vi "CRYAPI Spliter Ref.vi"(0 "VI Refnum":refnum<vi>) -> (1 "Left/Upper":refnum<vi>, 2 "Right/Lower":refnum<vi>)   [LabVIEW 2013]
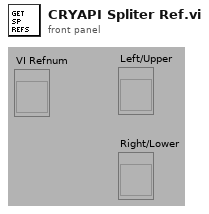
[diagram p1: front panel]
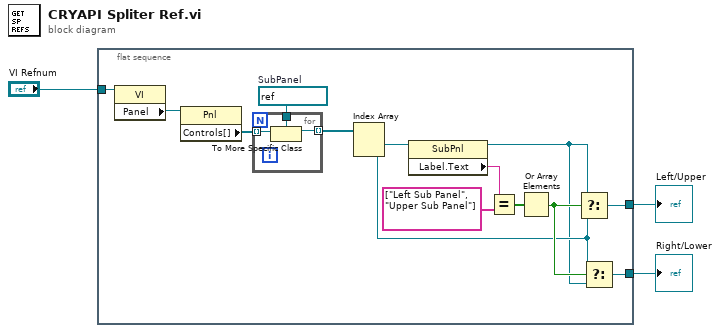
[diagram p0: block diagram]
diagram:
  n1 = flat-sequence {
    tunnel: "VI Refnum" -> [w17]
    tunnel: [w8] -> w2
    tunnel: [w7] -> w3
    frame #0 {
      w14 = refnum<vi> refnum  # SubPanel
      n2 = property class="VI"(reference=w17) -> ("Panel"=w16:refnum<vi>)  [unwired: 1 in, 2 out]
      n3 = property class="Pnl"(reference=w16) -> ("Controls[]"=w15:refnum<vi>[])  [unwired: 1 in, 2 out]
      n4 = for {
        tunnel: w15 -> [w20] mode=indexing
        tunnel: w14 -> [w19]
        tunnel: [w18] -> w13 mode=indexing
        n5 = To More Specific Class(target class=w19, reference=w20) -> (specific class reference=w18:refnum<vi>)  [unwired: 1 in, 1 out]
      }
      n6 = Index Array(array=w13) -> (element #1=w12:refnum<vi>, element #2=w5:refnum<vi>)  [unwired: 2 in]
      n7 = property class="SubPnl"(reference=w12) -> (reference out=w4:refnum<vi>, "Label.Text"=w11:string)  [unwired: 1 in, 1 out]
      n8 = Equal?(x=w11, y=string[] ["Left Sub Panel", "Upper Sub Panel"]) -> (x = y?=w9:bool[])
      n9 = Or Array Elements(Boolean array=w9) -> (logical OR=w6:bool)
      n10 = Select(t=w4, s=w6, f=w5) -> (s? t:f=w8:refnum<vi>)
      n11 = Select(t=w5, s=w6, f=w4) -> (s? t:f=w7:refnum<vi>)
    }
  }
  "Right/Lower" <- w3
  "Left/Upper" <- w2
